vi "Incomming Array Handler.vi"() -> ()   [LabVIEW 2016]
panel:
  in  "Ring":u16(ring)
  in  "Array":dbl[](array[numeric])
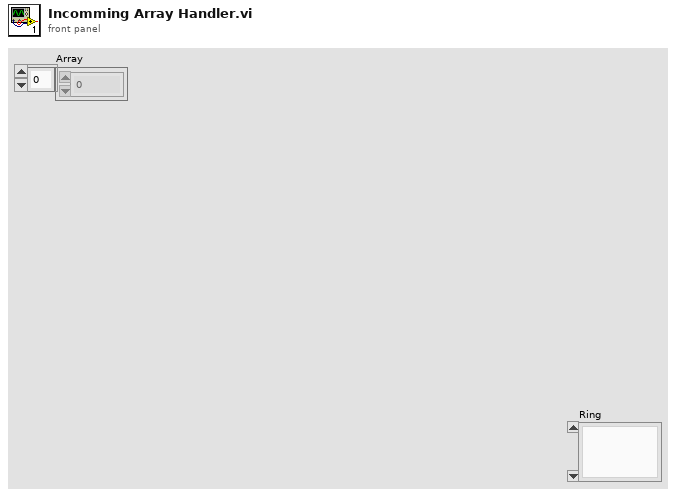
[diagram p1: front panel]
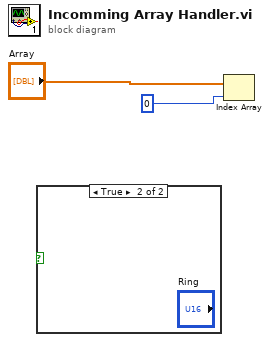
[diagram p0: block diagram]
diagram:
  n1 = case shown="True" {
    selector: _ -> [_ _]
    frame False {
    }
    frame True {
    }
  }
  n2 = Index Array(array="Array", index=0) -> (element=w1:dbl)
